vi "Begin.vi"(8 "error in (no error)":errorcluster, 10 "Configuration In":variant, 11 "Control Panel in":refnum<class "Control Panel.lvclass">) -> (0 "error out":errorcluster, 3 "Control Panel out":refnum<class "Control Panel.lvclass">)   [LabVIEW 2019, in "Control Panel.lvlib" / "Control Panel.lvclass"]
uses:
  Control Panel.lvclass
  <vilib>/Rock Robotics/SystemInterfaces/i2clib/i2c_bus.ctl
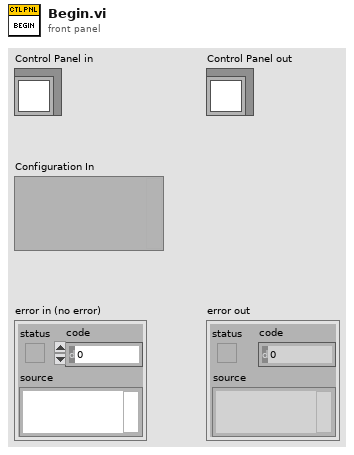
[diagram p1: front panel]
types:
  T1 = typedef "i2c_bus.ctl" = enum16{"I2C On-Board", "I2C MXP", "Invalid"}
  T2 = typedef "WPI_MotorControlDeviceRef.ctl" = cluster{"DeviceStatus":errorcluster, "Type":T3, "PWM":cluster{"PWM Channel":T4, "DeadBand":T5}, "CAN":cluster{"Device Number":u8, "SetOutput VI Ref":variant, "GetOutput VI Ref":variant, "Enable VI Ref":variant, "Disable VI Ref":variant, "Data":variant}, "Invert":bool, "DIO PWM":cluster{"PWM \"Enable\" Channel":T4, "DIOChannel":T6, "PWM Rate":dbl}}
  T3 = typedef "WPI_MotorControlType.ctl" = enum16{"PWM", "CAN", "DIO PWM"}
  T4 = typedef "FPGA_DIOPWMChannel.ctl" = enum8{"PWM 0", "PWM 1", "PWM 2", "PWM 3", "PWM 4", "PWM 5", "PWM 6", "PWM 7", "PWM 8", "PWM 9", "PWM MXP 0", "PWM MXP 1", "PWM MXP 2", "PWM MXP 3", "PWM MXP 4", "PWM MXP 5", "PWM MXP 6", "PWM MXP 7", "PWM MXP 8", "PWM MXP 9", "Invalid"}
  T5 = typedef "WPI_PWMDeadband.ctl" = cluster{"Name":string, "maxPositivePwm":i32, "minPositivePwm":i32, "centerPwm":i32, "maxNegativePwm":i32, "minNegativePwm":i32, "angularRange":u16}
  T6 = typedef "FPGA_DIOChannel.ctl" = enum8{"DIO 0", "DIO 1", "DIO 2", "DIO 3", "DIO 4", "DIO 5", "DIO 6", "DIO 7", "DIO 8", "DIO 9", "DIO MXP 0", "DIO MXP 1", "DIO MXP 2", "DIO MXP 3", "DIO MXP 4", "DIO MXP 5", "DIO MXP 6", "DIO MXP 7", "DIO MXP 8", "DIO MXP 9", "DIO MXP 10", "DIO MXP 11", "DIO MXP 12", "DIO MXP 13", "DIO MXP 14", "DIO MXP 15", "SPI Port CS1", "SPI Port CS2", "SPI Port CS3", "SPI Port MISO", "SPI Port MOSI", "Invalid"}
  T7 = typedef "Color Sensor V3 DevRef.ctl" = cluster{"I2CDevRef":T8}
  T8 = typedef "WPI_I2CDevRef.ctl" = cluster{"DevStatus":errorcluster, "Device Address":u8, "Handle":i32, "I2C Bus":T1}
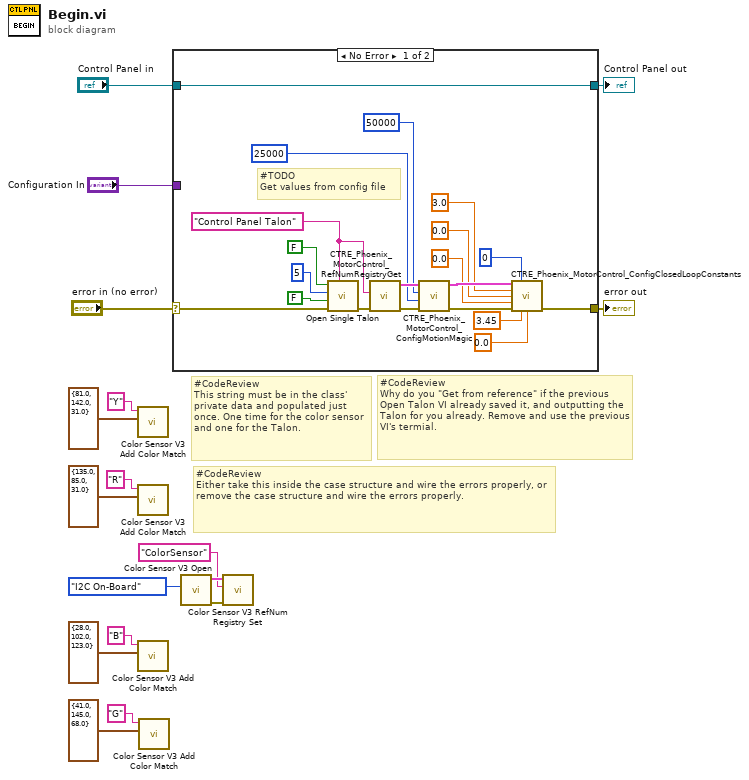
[diagram p0: block diagram]
diagram:
  # "#CodeReview\nWhy do you \"Get from reference\" if the previous Open Talon VI already saved it, and outputting the Talon for you already. Remove and use the previous VI's termial."
  # "#CodeReview\nThis string must be in the class' private data and populated just once. One time for the color sensor and one for the Talon."
  # "#CodeReview\nEither take this inside the case structure and wire the errors properly, or remove the case structure and wire the errors properly."
  n1 = call <vilib>:"Color Sensor V3 Add Color Match.vi"("Color"=cluster{"R":dbl, "G":dbl, "B":dbl} {"R"=81.0, "G"=142.0, "B"=31.0}, "Name"="Y") -> ()  [unwired: 10 in]
  n2 = call <vilib>:"Color Sensor V3 Add Color Match.vi"("Color"=cluster{"R":dbl, "G":dbl, "B":dbl} {"R"=135.0, "G"=85.0, "B"=31.0}, "Name"="R") -> ()  [unwired: 10 in]
  n3 = call <vilib>:"Color Sensor V3 Add Color Match.vi"("Color"=cluster{"R":dbl, "G":dbl, "B":dbl} {"R"=28.0, "G"=102.0, "B"=123.0}, "Name"="B") -> ()  [unwired: 10 in]
  n4 = call <vilib>:"Color Sensor V3 Add Color Match.vi"("Color"=cluster{"R":dbl, "G":dbl, "B":dbl} {"R"=41.0, "G"=145.0, "B"=68.0}, "Name"="G") -> ()  [unwired: 10 in]
  n5 = case shown="No Error" "error in (no error)" {
    selector: "error in (no error)" -> [w37 w39]
    tunnel: [w21 w39] -> w16
    tunnel: "Control Panel in" -> [w33 w38]
    tunnel: [w33 w38] -> w14
    tunnel: "Configuration In" -> [_ _]
    frame No Error {
      w18 = "Control Panel Talon"
      # "#TODO\nGet values from config file"
      n6 = call "Open Single Talon.vi"("refnum name"=w18, "error in (no error)"=w37, "sensor phase"=FALSE, "can id"=5, "invert"=FALSE) -> ("error out"=w30:errorcluster)  [unwired: 5 in, 1 out]
      n7 = call <vilib>:"CTRE_Phoenix_MotorControl_RefNumRegistryGet.vi"("error in (no error)"=w30, "refnum name"=w18) -> ("error out"=w29:errorcluster, "PhoenixMotorControlDevRef"=w32:T2)  [unwired: 8 in]
      n8 = call <vilib>:"CTRE_Phoenix_MotorControl_ConfigMotionMagic.vi"("error in (no error)"=w29, "Acceleration"=25000, "Cruise Velocity"=50000, "PhoenixMotorControlDevRef"=w32) -> ("error out"=w28:errorcluster, "PhoenixMotorControlDevRef"=w31:T2)  [unwired: 6 in]
      n9 = call <vilib>:"CTRE_Phoenix_MotorControl_ConfigClosedLoopConstants.vi"("PhoenixMotorControlDevRef"=w31, "slotIdx"=0, "P"=3.0, "I"=0.0, "D"=0.0, "error in (no error)"=w28, "F"=3.45, "I Zone"=0.0) -> ("error out"=w21:errorcluster)  [unwired: 6 in, 1 out]
    }
    frame Error {
    }
  }
  "error out" <- w16
  "Control Panel out" <- w14
  n10 = call <vilib>:"Color Sensor V3 Open.vi"("I2C Bus"=i2c_bus."I2C On-Board") -> ("error out"=w12:errorcluster, "ColorSensorDevRef"=w11:T7)  [unwired: 9 in]
  n11 = call <vilib>:"Color Sensor V3 RefNum Registry Set.vi"("error in (no error)"=w12, "refnum name"="ColorSensor", "ColorSensorDevRef"=w11) -> ()  [unwired: 7 in, 2 out]
